vi "readFromXML.vi"(8 "error in (no error)":errorcluster, 10 "XML in":string, 11 "PointingFileCommands in":refnum<class "PointingFileCommands.lvclass">) -> (0 "error out":errorcluster, 3 "PointingFileCommands out":refnum<class "PointingFileCommands.lvclass">)   [LabVIEW 2022 SP3, in "TCSDataDefinitions.lvlib" / "TCSCommand.lvlib" / "PointingFileCommands.lvlib" / "PointingFileCommands.lvclass"]
uses:
  PointingFileCommands.lvclass
  TCSTcsCommand/TCSTcsCommand.lvclass
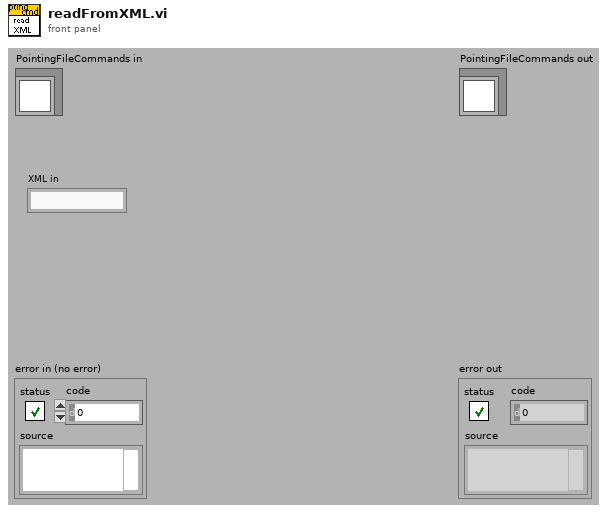
[diagram p1: front panel]
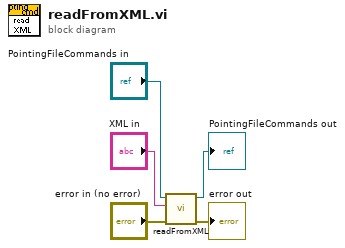
[diagram p0: block diagram]
diagram:
  n1 = call-parent "readFromXML.vi"("error in (no error)"="error in (no error)", "XMLin"="XML in", "TCSTcsCommand in"="PointingFileCommands in") -> ("error out"=→"error out":errorcluster, "TCSTcsCommand out"=→"PointingFileCommands out":refnum<class "PointingFileCommands.lvclass">)  [unwired: 7 out]
